vi "Read Messenger Reference.vi"(8 "error in (no error)":errorcluster, 11 "Composite Task in":refnum<class "Linked List Task.lvclass">) -> (0 "error out":errorcluster, 2 "Messenger Reference":refnum<data-value>, 3 "Composite Task out":refnum<class "Linked List Task.lvclass">)   [LabVIEW 2024, in "Linked List Task.lvclass"]
uses:
  Linked List Task.lvclass
  Linked List Task.lvclass/Linked List Task.ctl
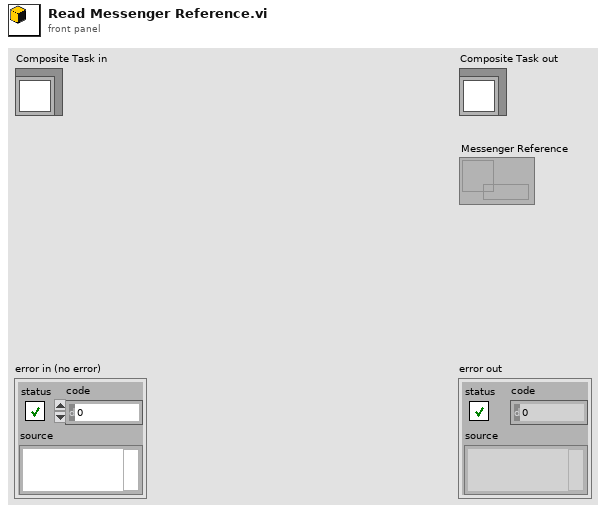
[diagram p1: front panel]
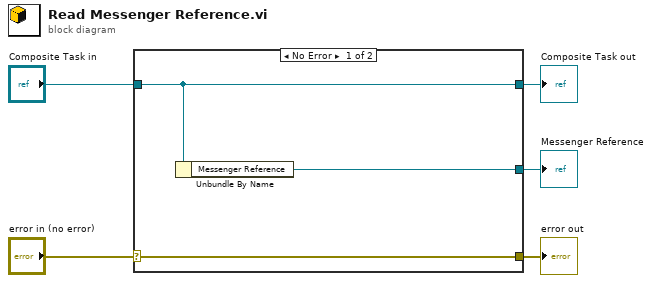
[diagram p0: block diagram]
diagram:
  n1 = case shown="No Error" "error in (no error)" {
    selector: "error in (no error)" -> [w8 w9]
    tunnel: [w8 w9] -> w4
    tunnel: [w7 w10] -> w2
    tunnel: "Composite Task in" -> [w7 w10]
    tunnel: [w6 _] -> w1
    frame No Error {
      n2 = Unbundle By Name(w7) -> ("Messenger Reference"=w6:refnum<data-value>)
    }
    frame Error {
    }
  }
  "error out" <- w4
  "Composite Task out" <- w2
  "Messenger Reference" <- w1
